vi "Move Window.vi"(8 "error in (no error)":errorcluster, 10 "window position":cluster{"Left":i16, "Top":i16}, 11 "VI Ref":refnum<vi>) -> (0 "error out":errorcluster)   [LabVIEW 2019, in "DSF Core.lvlib" / "Thread.lvclass"]
uses:
  Thread.lvclass
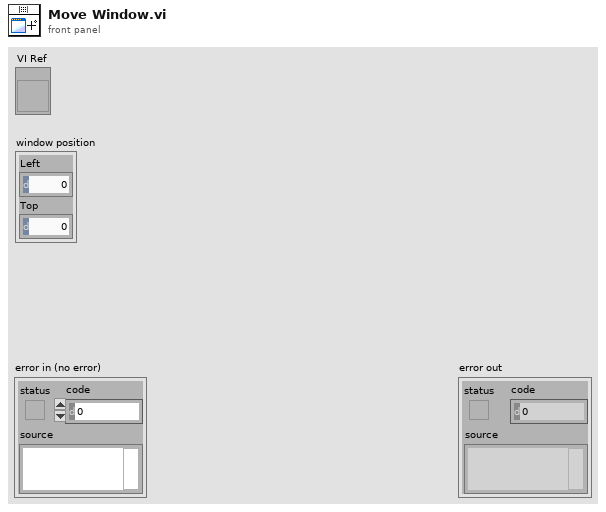
[diagram p1: front panel]
types:
  T1 = typedef "LVRectTypeDef.ctl" = cluster{"Left":i16, "Top":i16, "Right":i16, "Bottom":i16}
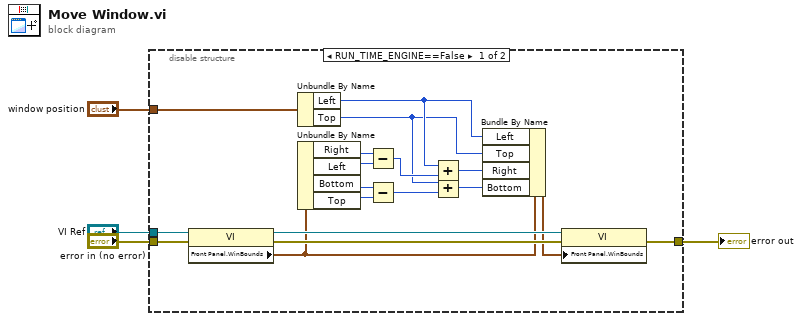
[diagram p0: block diagram]
diagram:
  n1 = disable-structure shown="RUN_TIME_ENGINE==False" {
    disable-tunnel: "error in (no error)" -> [w11 w23]
    disable-tunnel: "window position" -> [w10 _]
    disable-tunnel: "VI Ref" -> [w9 _]
    disable-tunnel: [w5 w23] -> w1
    frame condition #0 (active) {
      n2 = property class="VI"(reference=w9, error in=w11) -> (reference out=w8:refnum<vi>, error out=w12:errorcluster, "Front Panel.WinBounds"=w6:T1)
      n3 = Unbundle By Name(w10) -> ("Left"=w18:i16, "Top"=w15:i16)
      n4 = Unbundle By Name(w6) -> ("Right"=w22:i16, "Left"=w21:i16, "Bottom"=w20:i16, "Top"=w19:i16)
      n5 = Subtract(x=w22, y=w21) -> (x-y=w16:i16)
      n6 = Subtract(x=w20, y=w19) -> (x-y=w13:i16)
      n7 = Add(x=w18, y=w16) -> (x+y=w17:i16)
      n8 = Add(x=w15, y=w13) -> (x+y=w14:i16)
      n9 = Bundle By Name(cluster=w6, "Left"=w18, "Top"=w15, "Right"=w17, "Bottom"=w14) -> (w7:T1)
      n10 = property class="VI"(reference=w8, error in=w12, "Front Panel.WinBounds"=w7) -> (error out=w5:errorcluster)  [unwired: 1 out]
    }
    frame condition #1 {
    }
  }
  "error out" <- w1
